vi "LabelPriv.vi"(4 "Label Properties":T1={"Text"={"Color"=2147483647, "Background Color"=2147483647, "Font Size (points)"=0, "Font Style"=enum."Automatic", "Rotation Angle"=nan}} {"Text"."Background Color" items=["Automatic"=2147483647, "Black"=0, "White"=16777215, "Red"=16711680, "Green"=2263842, "Blue"=255, "Cyan"=65535, "Magenta"=16711935, "Yellow"=16776960]; "Text"."Font Size (points)" items=["Automatic"=0, "XX-Small"=-1, "X-Small"=-2, "Small"=-3, "Medium"=-4, "Large"=-5, "X-Large"=-6, "XX-Large"=-7]; "Text"."Color" items=["Automatic"=2147483647, "Black"=0, "White"=16777215, "Red"=16711680, "Green"=2263842, "Blue"=255, "Cyan"=65535, "Magenta"=16711935, "Yellow"=16776960]}, 7 "Location":T6(ring), 8 "error in (no error)":errorcluster, 10 "Label":string, 11 "Plot ID":T7 format="%x") -> (0 "error out":errorcluster)   [LabVIEW 2013, in "Advanced Plotting Toolkit.lvlib"]
uses:
  Advanced Plotting Toolkit.lvlib
  typedefs/PlotID.ctl
  LabelProperties.ctl
  properties/Text.ctl
  typedefs/PlotColor.ctl
  properties/Text_FontSize.ctl
  properties/Text_FontStyle.ctl
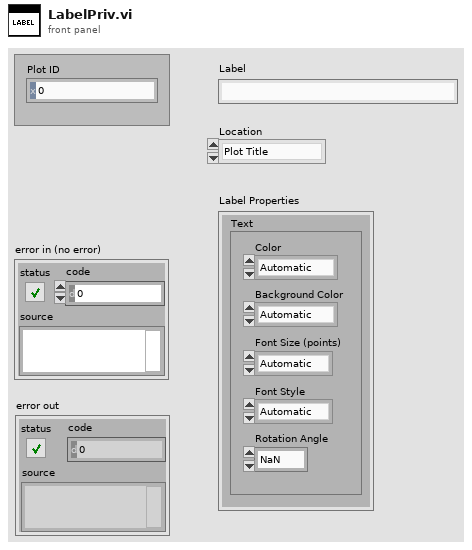
[diagram p1: front panel]
types:
  T1 = typedef "Advanced Plotting Toolkit.lvlib/LabelProperties.ctl" = cluster{"Text":T2}
  T2 = typedef "Advanced Plotting Toolkit.lvlib/Text.ctl" = cluster{"Color":T3, "Background Color":T3, "Font Size (points)":T4, "Font Style":T5, "Rotation Angle":dbl}
  T3 = typedef "Advanced Plotting Toolkit.lvlib/PlotColor.ctl" = u32
  T4 = typedef "Advanced Plotting Toolkit.lvlib/Text_FontSize.ctl" = i32
  T5 = typedef "Advanced Plotting Toolkit.lvlib/Text_FontStyle.ctl" = enum16{"Automatic", "Normal", "Italic", "Bold"}
  T6 = enum16{"Plot Title", "X Axis Label", "Y Axis Label"}
  T7 = typedef "Advanced Plotting Toolkit.lvlib/PlotID.ctl" = i32
  T8 = typedef "Advanced Plotting Toolkit.lvlib/KeyValue.ctl" = cluster{"Key":string, "Value":string}
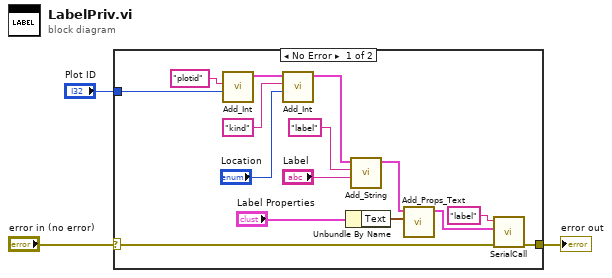
[diagram p0: block diagram]
diagram:
  n1 = case shown="No Error" "error in (no error)" {
    selector: "error in (no error)" -> [w11 w19]
    tunnel: "Plot ID" -> [w18 _]
    tunnel: [w10 w19] -> w1
    frame No Error {
      n2 = call "Add_Int.vi"("Value"=w18, "Key"="plotid") -> ("Keyword Array Out"=w7:T8[])  [unwired: 9 in]
      n3 = call "Add_Int.vi"("Value"="Location", "Key"="kind", "Keyword Array"=w7) -> ("Keyword Array Out"=w6:T8[])  [unwired: 8 in]
      n4 = Unbundle By Name("Label Properties") -> ("Text"=w4:T2)
      n5 = call "Add_String.vi"("Value"="Label", "Key"="label", "Keyword Array"=w6) -> ("Keyword Array Out"=w14:T8[])  [unwired: 8 in]
      n6 = call "Add_Props_Text.vi"("Text Properties"=w4, "Keyword Array"=w14) -> ("Keyword Array Out"=w13:T8[])  [unwired: 9 in]
      n7 = call "SerialCall.vi"("error in (no error)"=w11, "data"=w13, "Resource"="label") -> ("error out"=w10:errorcluster)  [unwired: 7 in, 1 out]
    }
    frame Error {
    }
  }
  "error out" <- w1
